vi "Init.vi"(0 "I2C Ref In":T1={"myRIO Reference"={"myRIO Model"=enum."Unknown", "myRIO Hardware Reference"={"Generic FPGA Reference"=refnum, "Allow multiple opens"=FALSE}}, "I2C Channels Enum"=enum."Not Connected", "I2C Configuration"={"I2C Transfer Rate"=enum."Fast mode (400 kbps)"}}, 1 "Accel Full Scale Range":T10, 2 "Gyro Full Scale Range":T9, 5 "Device Address":T11=104 items=["0x68"=104, "0x69"=105], 9 "Clock Source":u8=1, 11 "error in (no error)":errorcluster) -> (4 "I2C Ref Out":T1={"myRIO Reference"={"myRIO Model"=enum."Unknown", "myRIO Hardware Reference"={"Generic FPGA Reference"=refnum, "Allow multiple opens"=FALSE}}, "I2C Channels Enum"=enum."Not Connected", "I2C Configuration"={"I2C Transfer Rate"=enum."Fast mode (400 kbps)"}}, 15 "error out":errorcluster)   [LabVIEW 2016]
uses:
  DeviceAddresses.ctl
  LIFA MPU-60X0 LV9/AccelFullScaleRanges.ctl
  LIFA MPU-60X0 LV9/GyroFullScaleRanges.ctl
  <vilib>/myRIO/Instrument Drivers/Onboard IO/I2C/typedefs/I2C Reference.ctl
  <vilib>/myRIO/Common/Instrument Driver Framework/Utilities/typedefs/myRIO Generic Hardware Reference.ctl
  <vilib>/myRIO/Common/Instrument Driver Framework/Utilities/typedefs/Hardware Version Enum.ctl
  <vilib>/myRIO/Common/Instrument Driver Framework/Utilities/typedefs/myRIO v1.0 Reference.ctl
  <vilib>/myRIO/Common/Instrument Driver Framework/Utilities/typedefs/Generic FPGA Reference.ctl
  <vilib>/myRIO/Common/Instrument Driver Framework/myRIO v1.0/I2C/typedefs/I2C Channels Enum.ctl
  <vilib>/myRIO/Instrument Drivers/Onboard IO/I2C/typedefs/I2C Configuration.ctl
  <vilib>/myRIO/Instrument Drivers/Onboard IO/I2C/typedefs/I2C Transfer Rate.ctl
  LIFA MPU-60X0 LV9/LIFA MPU-60X0.lvlib
  <vilib>/myRIO/Instrument Drivers/Onboard IO/I2C/I2C.lvlib
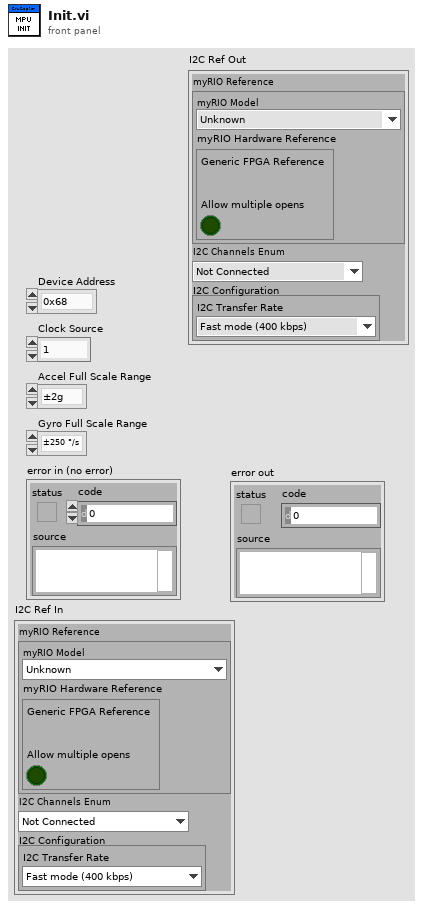
[diagram p1: front panel]
types:
  T1 = typedef "I2C.lvlib/I2C Reference.ctl" = cluster{"myRIO Reference":T2, "I2C Channels Enum":T6, "I2C Configuration":T7}
  T2 = typedef "myRIO Generic Hardware Reference.ctl" = cluster{"myRIO Model":T3, "myRIO Hardware Reference":T4}
  T3 = typedef "Hardware Version Enum.ctl" = enum16{"Unknown", "myRIO-1900", "myRIO-1950", "roboRIO", "NI ELVIS RIO CM"}
  T4 = typedef "myRIO v1.0 Reference.ctl" = cluster{"Generic FPGA Reference":T5, "Allow multiple opens":bool}
  T5 = typedef "Generic FPGA Reference.ctl" = refnum<k20>
  T6 = typedef "I2C Channels Enum.ctl" = enum16{"Not Connected", "A/I2C", "B/I2C", "I2C/I2C"}
  T7 = typedef "I2C.lvlib/I2C Configuration.ctl" = cluster{"I2C Transfer Rate":T8}
  T8 = typedef "I2C.lvlib/I2C Transfer Rate.ctl" = enum16{"Standard mode (100 kbps)", "Fast mode (400 kbps)"}
  T9 = typedef "LIFA MPU-60X0.lvlib/GyroFullScaleRanges.ctl" = enum8{"±250 °/s", "±500 °/s", "±1000 °/s", "±2000 °/s"}
  T10 = typedef "LIFA MPU-60X0.lvlib/AccelFullScaleRanges.ctl" = enum16{"±2g", "±4g", "±8g", "±16g"}
  T11 = typedef "DeviceAddresses.ctl" = u8
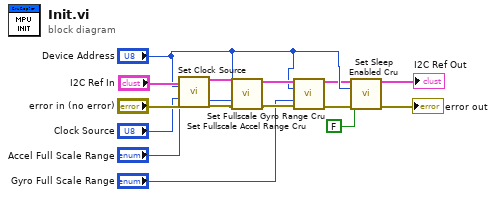
[diagram p0: block diagram]
diagram:
  n1 = call "Set Clock Source.vi"("I2C Ref In"="I2C Ref In", "Device Address"="Device Address", "Clock Source"="Clock Source", "error in (no error)"="error in (no error)") -> ("I2C Ref Out"=w10:T1, "error out"=w12:errorcluster)  [unwired: 10 in]
  n2 = call "Set Fullscale Accel Range Cru.vi"("I2C Ref In"=w10, "Device Address"="Device Address", "Accel Full Scale Range"="Accel Full Scale Range", "error in (no error)"=w12) -> ("I2C Ref Out"=w9:T1, "error out"=w8:errorcluster)  [unwired: 10 in]
  n3 = call "Set Fullscale Gyro Range Cru.vi"("I2C Ref In"=w9, "Device Address"="Device Address", "Gyro Full Scale Range"="Gyro Full Scale Range", "error in (no error)"=w8) -> ("I2C Ref Out"=w4:T1, "error out"=w3:errorcluster)  [unwired: 10 in]
  n4 = call "Set Sleep Enabled Cru.vi"("I2C Ref In"=w4, "Device Address"="Device Address", "Sleep?"=FALSE, "error in (no error)"=w3) -> ("I2C Ref Out"=→"I2C Ref Out":T1, "error out"=→"error out":errorcluster)  [unwired: 10 in]
